vi "sim.vi"() -> ()   [LabVIEW 2021]
uses:
  <vilib>/Math Plots/2D Math Plots/2D Compass/2D Compass XCtrl/2D Compass.xctl
  <vilib>/Math Plots/2D Math Plots/2D Compass/2D Compass Datatype/Public/Plot Helper (Vector).vi
  <vilib>/Math Plots/2D Math Plots/2D Compass/2D Compass Datatype/2D Compass Datatype.lvclass
panel:
  out "Heading speed":sgl
  out "Speed":sgl
  out "heading":sgl
  out "Iskele SP":i16(slide) scale=-100.0..100.0
  out "Sancak SP":i16(slide) scale=-100.0..100.0
  in  "Sapma":i16(slide) scale=-200.0..200.0
  out "check":i32
  out "Heading":refnum<class "2D Plot Datatype.lvclass">[](xcontrol) caption="2D Compass 2"
  in  "History Data":i32=5
  out "Speed":dbl(knob) scale=0.0..3.0
  out "XY Graph":cluster{sgl[], sgl[]}(graph)
  in  "Senkron":bool
  in  "Iskele RPM indicator":i16(slide) scale=0.0..100.0
  in  "Sancak RPM indicator":i16(slide) scale=0.0..100.0
  out "Sancak RPM":cluster{"Numeric 3":dbl, "Numeric 3":dbl}(knob) scale=-100.0..100.0
  out "Iskele RPM":cluster{"Numeric 3":dbl, "Numeric 3":dbl}(knob)={"Numeric 3"=0.0, "Numeric 3"=-50.33650220555203} scale=-100.0..100.0
  out "Eta":sgl[](array[numeric])
  out "Nu":sgl[](array[numeric])
  in  "stop":bool
  out "Numeric":i32
  out "Python path":path
  out "error out":errorcluster
  in  "error in (no error)":errorcluster
  # "Hiz kontrolü\nheading"
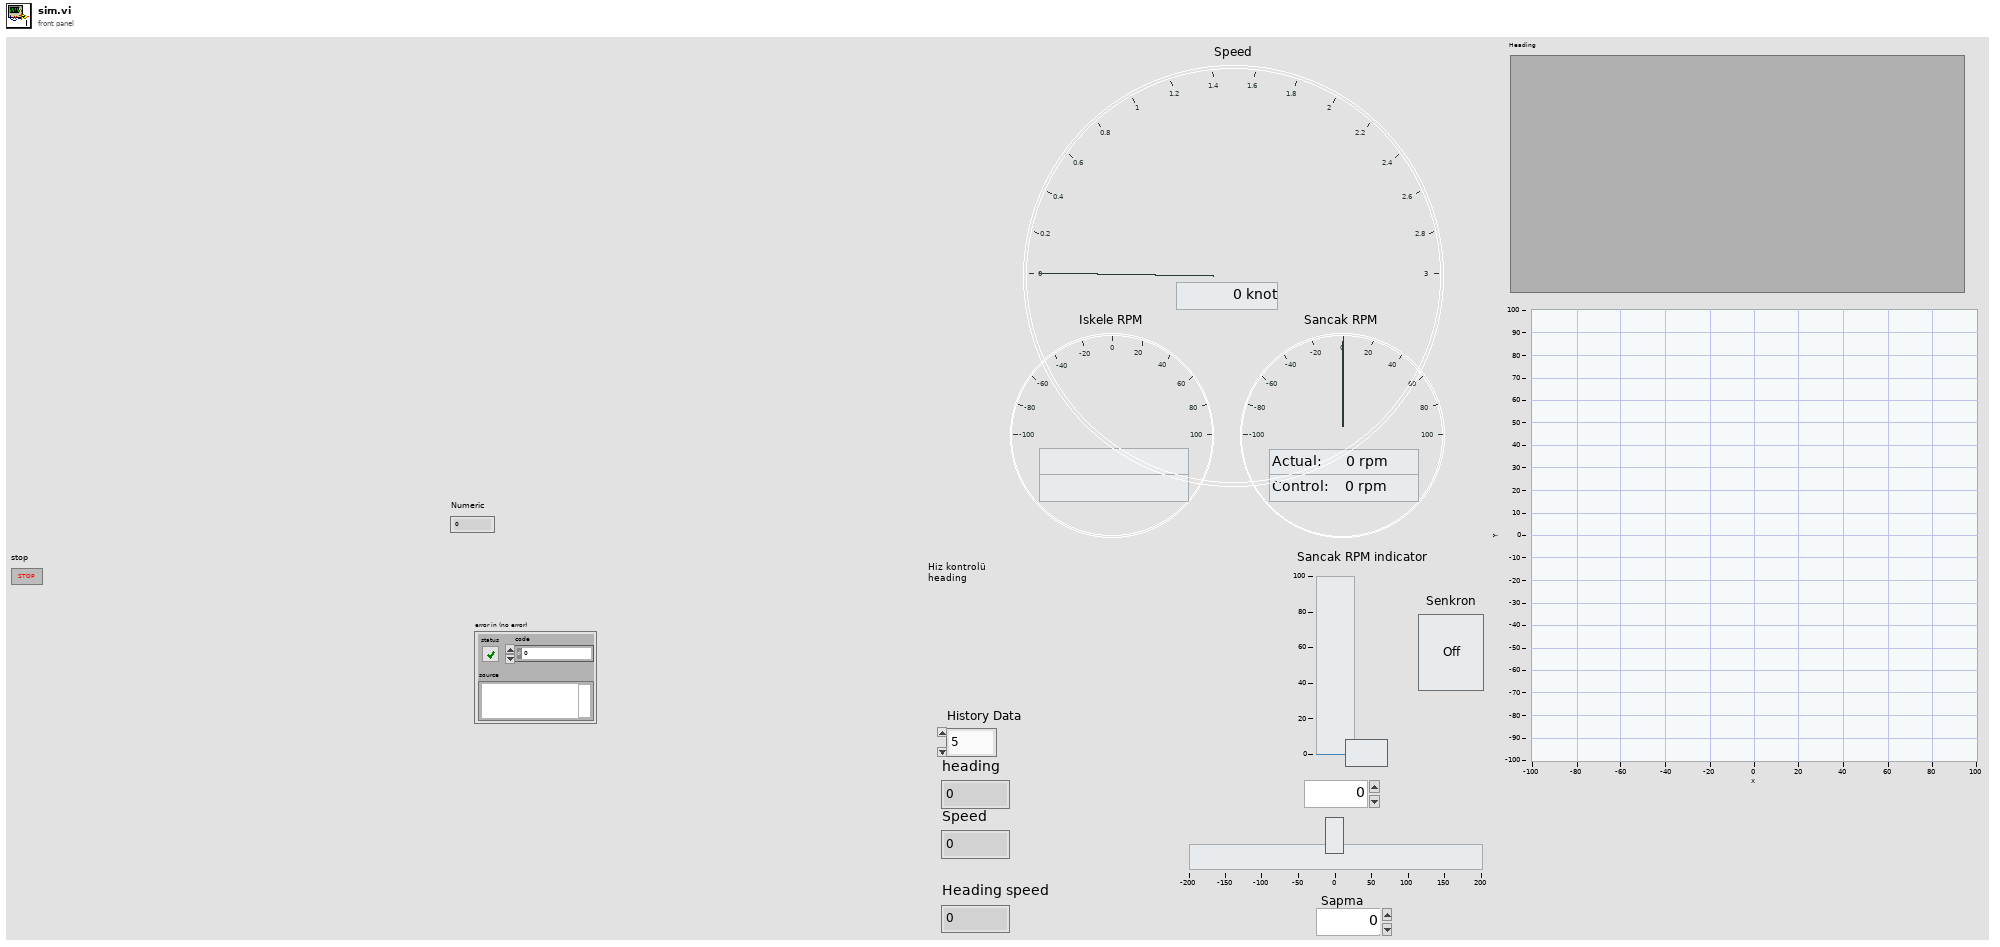
[diagram p1: front panel]
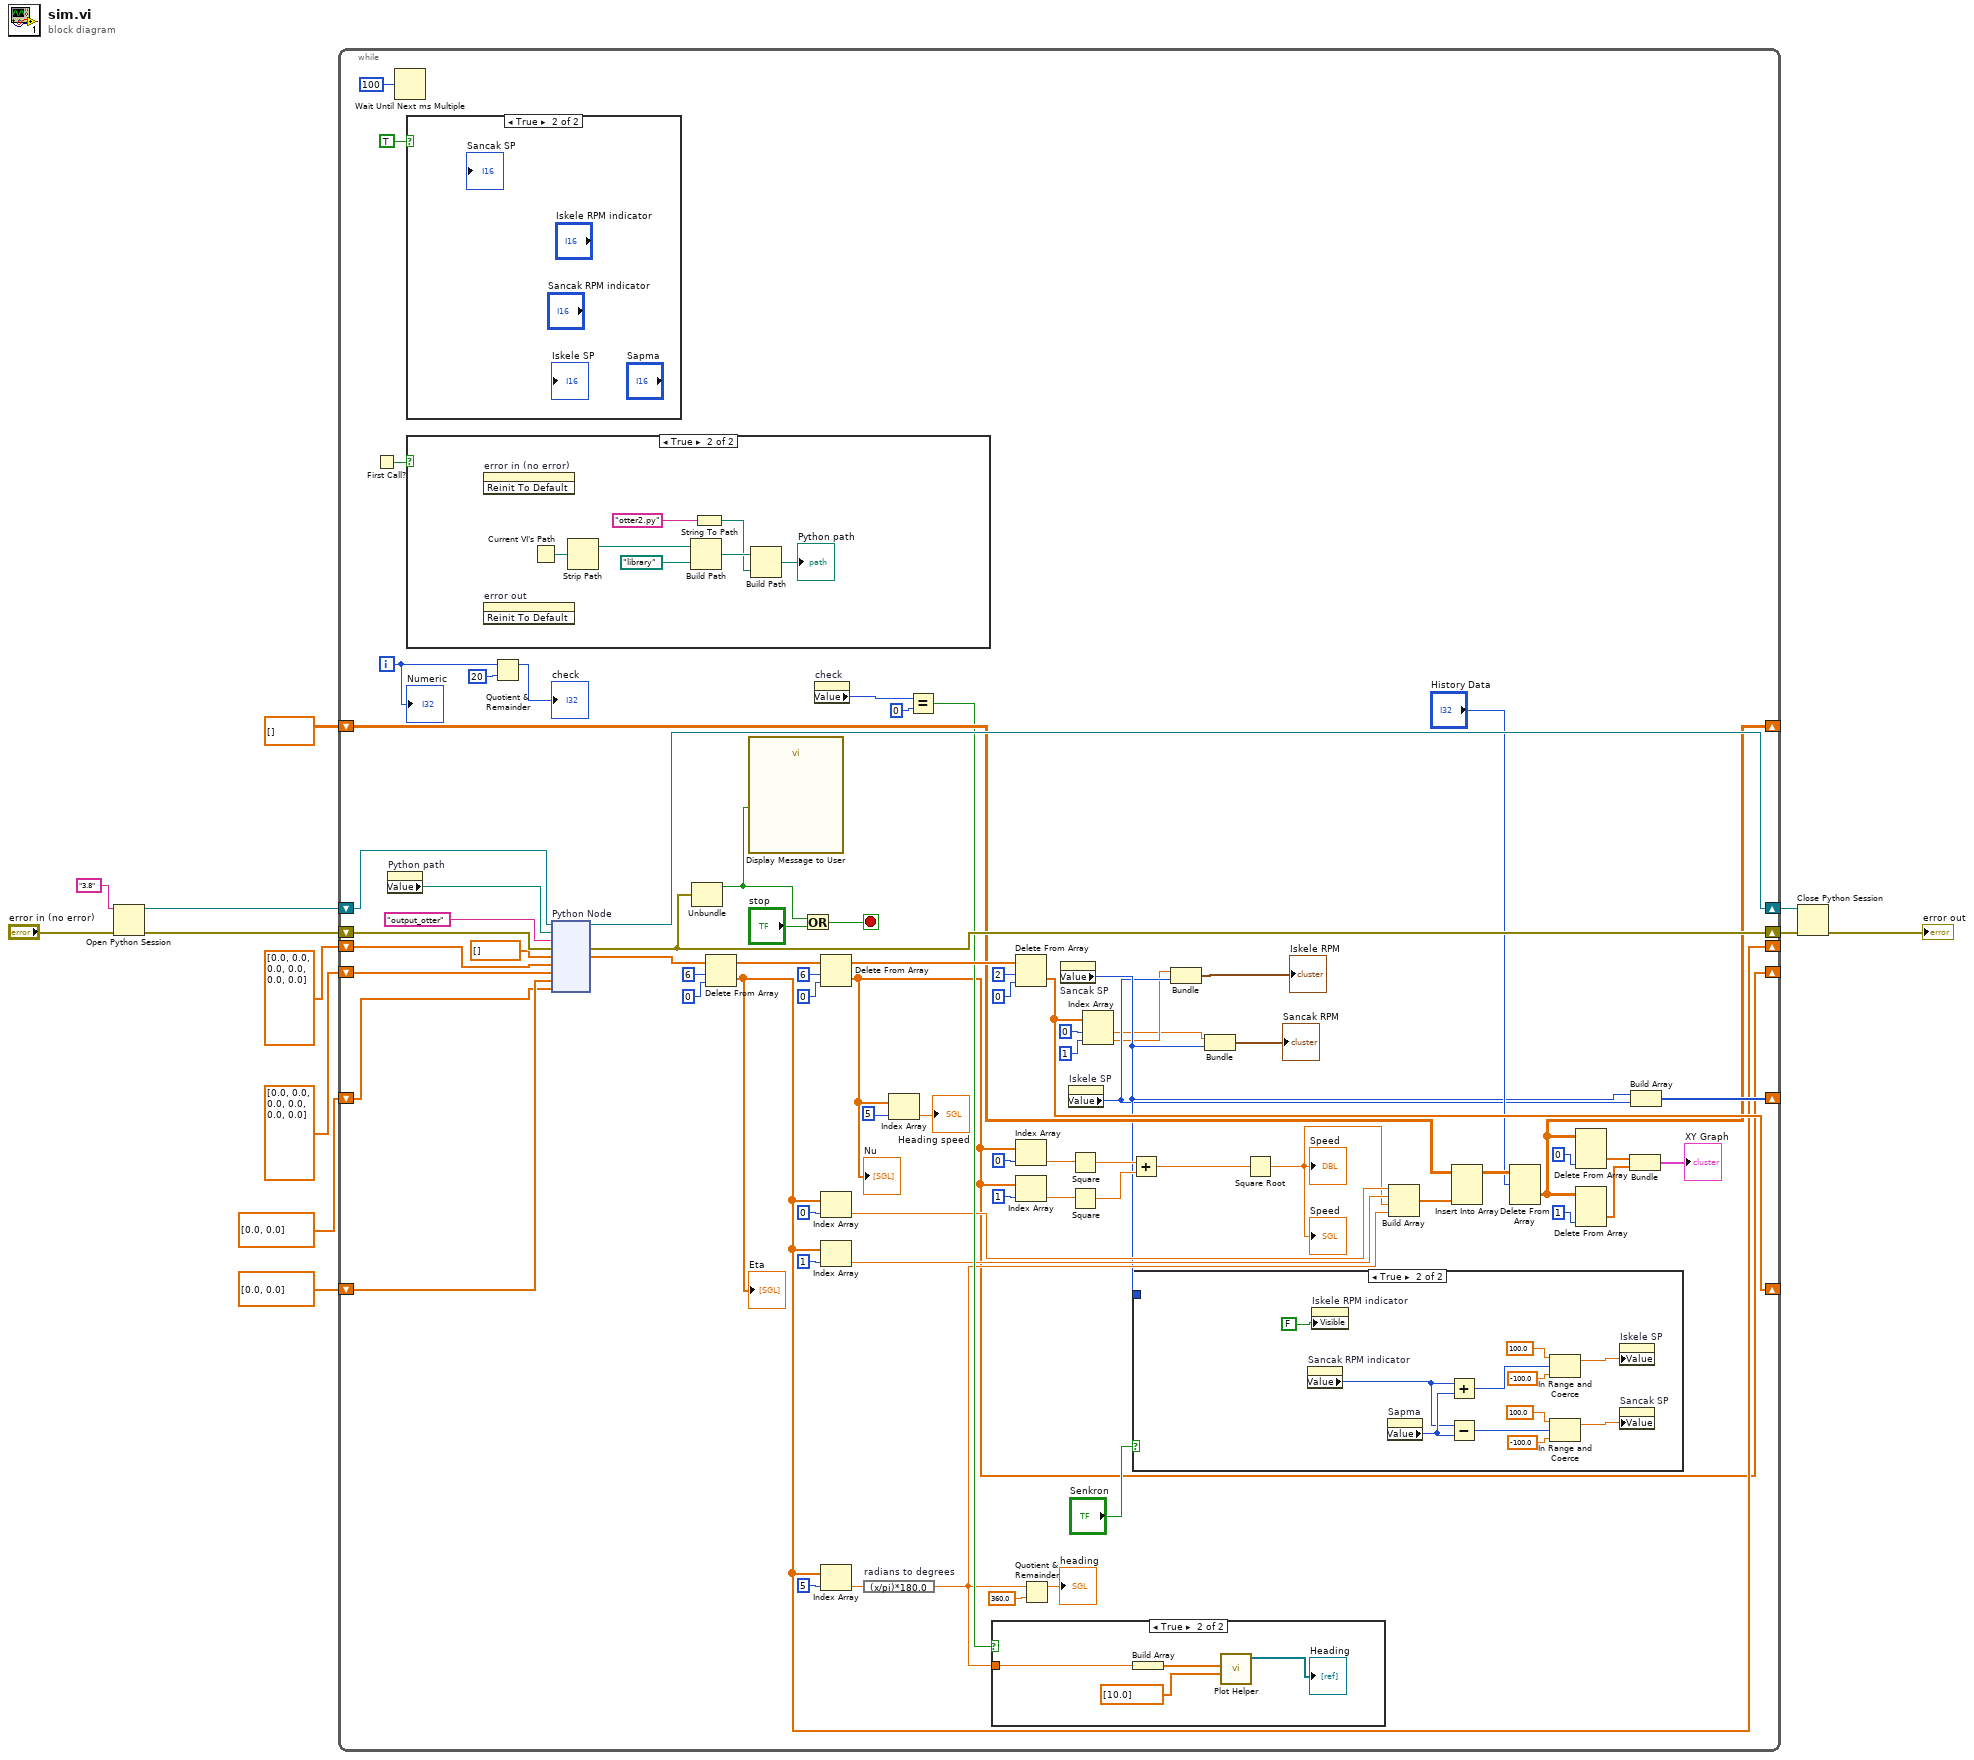
[diagram p0: block diagram]
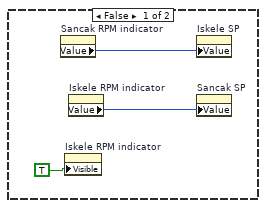
[diagram p4: hidden frame]
diagram:
  n1 = Open Python Session(python version="3.8" ("Python version"), 3:"error in (no error)") -> (session out=w9:refnum<k35>, error out=w11:errorcluster)  [unwired: 1 in]
  n2 = while {
    shift-right: [w80] -> w10
    shift-left: w11 -> [w86]
    shift-right: [w84] -> w8
    shift-left: w9 -> [w85]
    shift-right: [w46] -> _
    shift-left: sgl[] [0.0, 0.0, 0.0, 0.0, 0.0, 0.0] -> [w75]
    shift-right: [w15] -> _
    shift-left: sgl[] [0.0, 0.0, 0.0, 0.0, 0.0, 0.0] -> [w74]
    shift-right: [w60] -> _
    shift-left: sgl[] [0.0, 0.0] -> [w73]
    shift-right: [w71] -> _
    shift-left: sgl[] [0.0, 0.0] -> [w72]
    shift-right: [w35] -> _
    shift-left: sgl[][] [] -> [w44]
    i -> [w34]
    stop <- w78 stop-if-true
    n3 = First Call?() -> (First Call?: T/F=w81:bool)
    n4 = property on="Python path" class="Path"() -> ("Value"=w82:path)  [unwired: 2 in, 2 out]
    n5 = Wait Until Next ms Multiple(millisecond multiple=u32 100) -> ()  [unwired: 1 out]
    n6 = case shown="True" TRUE {
      frame False {
      }
      frame True {
      }
    }
    n7 = case shown="True" w81 {
      frame False {
      }
      frame True {
        n8 = invoke on="error in (no error)" class="Clust (strict)" method="Reinit To Default"() -> ()  [unwired: 3 in, 3 out]
        n9 = invoke on="error out" class="Clust (strict)" method="Reinit To Default"() -> ()  [unwired: 3 in, 3 out]
        n10 = Current VI's Path() -> (path=w107:path)
        n11 = Strip Path(path=w107) -> (stripped path=w110:path)  [unwired: 1 out]
        n12 = Build Path(base path=w110, name or relative path=path "library") -> (appended path=w109:path)
        n13 = String To Path(string="otter2.py") -> (path=w108:path)
        n14 = Build Path(base path=w109, name or relative path=w108) -> (appended path=→"Python path":path)
      }
    }
    n15 = Quotient & Remainder(x=w34, y=20) -> (x-y*floor(x/y)=→"check":i32)  [unwired: 1 out]
    n16 = node "Python Node"(w85, w82, "output_otter" ("function name"), w86, sgl[] [], w75, w74, w73, w72) -> (w84:refnum<k35>, w80:errorcluster, w70:sgl[])  [unwired: 4 in, 2 out]
    n17 = Unbundle(w80) -> ("status"=w77:bool)  [unwired: 2 out]
    n18 = Delete From Array(array=w70, length=6, index=0) -> (deleted portion=w46:sgl[], array with subset deleted=w65:sgl[])
    "Eta" <- w46
    n19 = call "Display Message to User"("Enable"=w77) -> ()  [unwired: 9 in, 2 out]
    n20 = Or(x=w77, y="stop") -> (x .or. y?=w78:bool)
    n21 = property on="check" class="DigNum (strict)"() -> ("Value"=w31:i32)  [unwired: 2 in, 2 out]
    n22 = Delete From Array(array=w65, length=6, index=0) -> (deleted portion=w15:sgl[], array with subset deleted=w62:sgl[])
    "Nu" <- w15
    n23 = Index Array(array=w46, index=0) -> (element=w23:sgl)
    n24 = Index Array(array=w46, index=1) -> (element=w24:sgl)
    n25 = Index Array(array=w46, index=5) -> (element=w36:sgl)
    n26 = expression code="(x/pi)*180.0" "radians to degrees"(w36) -> (w26:sgl)
    n27 = Index Array(array=w15, index=5) -> (element=→"Heading speed":sgl)
    n28 = Equal?(x=w31, y=0) -> (x = y?=w29:bool)
    n29 = case shown="True" w29 {
      tunnel: w26 -> [_ w88]
      frame False {
      }
      frame True {
        n30 = Build Array(w88) -> (w89:sgl[])
        n31 = call-poly <vilib>:"Plot Helper.vi"("radius vector"=dbl[] [10.0], "theta vector"=w89) -> ("2D Plot Class Obj Array out"=→"Heading":refnum<class "2D Plot Datatype.lvclass">[])  [unwired: 2 in, 7 out]
      }
    }
    n32 = Delete From Array(array=w62, length=2, index=0) -> (deleted portion=w60:sgl[])  [unwired: 1 out]
    n33 = Index Array(array=w15, index=0) -> (element=w49:sgl)
    n34 = Index Array(array=w15, index=1) -> (element=w50:sgl)
    n35 = Quotient & Remainder(x=w26, y=sgl 360.0) -> (x-y*floor(x/y)=→"heading":sgl)  [unwired: 1 out]
    n36 = property on="Sancak SP" class="Slide (strict)"() -> ("Value"=w19:i16)  [unwired: 2 in, 2 out]
    n37 = property on="Iskele SP" class="Slide (strict)"() -> ("Value"=w18:i16)  [unwired: 2 in, 2 out]
    n38 = Square(x=w49) -> (x^2=w20:sgl)
    n39 = Square(x=w50) -> (x^2=w22:sgl)
    n40 = Index Array(array=w60, index #1=0 ("index"), index #2=1 ("index")) -> (element #1=w16:sgl, element #2=w17:sgl)
    n41 = Add(x=w20, y=w22) -> (x+y=w48:sgl)
    n42 = case shown="True" "Senkron" {
      tunnel: w19 -> [_ _]
      frame False {
        n43 = property on="Sancak RPM indicator" class="Slide (strict)"() -> ("Value"=w93:i16)  [unwired: 2 in, 2 out]
        n44 = property on="Iskele RPM indicator" class="Slide (strict)"("Visible"=TRUE) -> ()  [unwired: 2 in, 2 out]
        n45 = property on="Iskele RPM indicator" class="Slide (strict)"() -> ("Value"=w92:i16)  [unwired: 2 in, 2 out]
        n46 = property on="Iskele SP" class="Slide (strict)"("Value"=w93) -> ()  [unwired: 2 in, 2 out]
        n47 = property on="Sancak SP" class="Slide (strict)"("Value"=w92) -> ()  [unwired: 2 in, 2 out]
      }
      frame True {
        n48 = property on="Sancak RPM indicator" class="Slide (strict)"() -> ("Value"=w95:i16)  [unwired: 2 in, 2 out]
        n49 = property on="Iskele RPM indicator" class="Slide (strict)"("Visible"=FALSE) -> ()  [unwired: 2 in, 2 out]
        n50 = property on="Sapma" class="Slide (strict)"() -> ("Value"=w104:i16)  [unwired: 2 in, 2 out]
        n51 = Add(x=w95, y=w104) -> (x+y=w97:i16)
        n52 = Subtract(x=w95, y=w104) -> (x-y=w101:i16)
        n53 = In Range and Coerce(upper limit=100.0, x=w97, lower limit=-100.0) -> (coerced(x)=w96:dbl)  [unwired: 1 out]
        n54 = In Range and Coerce(upper limit=100.0, x=w101, lower limit=-100.0) -> (coerced(x)=w100:dbl)  [unwired: 1 out]
        n55 = property on="Iskele SP" class="Slide (strict)"("Value"=w96) -> ()  [unwired: 2 in, 2 out]
        n56 = property on="Sancak SP" class="Slide (strict)"("Value"=w100) -> ()  [unwired: 2 in, 2 out]
      }
    }
    n57 = Bundle(w17, "Value"=w18) -> (→"Iskele RPM":cluster{sgl, "Value":i16})  [unwired: 1 in]
    n58 = Bundle(w16, "Value"=w19) -> (→"Sancak RPM":cluster{sgl, "Value":i16})  [unwired: 1 in]
    n59 = Square Root(x=w48) -> (sqrt(x)=w21:sgl)
    "Speed" <- w21
    "Speed" <- w21
    n60 = Build Array(w23, w24, w21, w26) -> (w43:sgl[])
    n61 = Insert Into Array(array=w44, new element=w43) -> (w42:sgl[][])  [unwired: 2 in]
    n62 = Delete From Array(array=w42, length="History Data") -> (deleted portion=w35:sgl[][])  [unwired: 2 in, 1 out]
    n63 = Delete From Array(array=w35, index (col)=0 ("disabled index (col)")) -> (deleted portion=w38:sgl[])  [unwired: 2 in, 1 out]
    n64 = Delete From Array(array=w35, index (col)=1 ("disabled index (col)")) -> (deleted portion=w37:sgl[])  [unwired: 2 in, 1 out]
    n65 = Bundle(w38, w37) -> (→"XY Graph":cluster{sgl[], sgl[]})  [unwired: 1 in]
    n66 = Build Array(w19, w18) -> (w71:i16[])
    "Numeric" <- w34
  }
  n67 = Close Python Session(session in=w8, error in=w10) -> (11:→"error out":errorcluster)
